vi "448benchmark1.vi"() -> ()   [LabVIEW 2017]
uses:
  user.lib/_NEVSTOP/Communicable State Machine(CSM)/_Support/Typedef/_CSM_GlobalLog_MSG.ctl
  user.lib/_NEVSTOP/Communicable State Machine(CSM)/_Support/Typedef/_CSM_Response Source Message.ctl
  user.lib/_NEVSTOP/Communicable State Machine(CSM)/_Support/Typedef/_CSM_GlobalLog_MSG_TYPE.ctl
  user.lib/_NEVSTOP/Communicable State Machine(CSM)/_Support/GlobalEvent/GEvt-Refs.ctl
  user.lib/_NEVSTOP/Communicable State Machine(CSM)/Communicable State Machine.lvlib
panel:
  out "inside 2":i32
  out "outside 2":i32
  out "inside":i32
  out "outside":i32
  out "unit (ms)":dbl[][](graph)
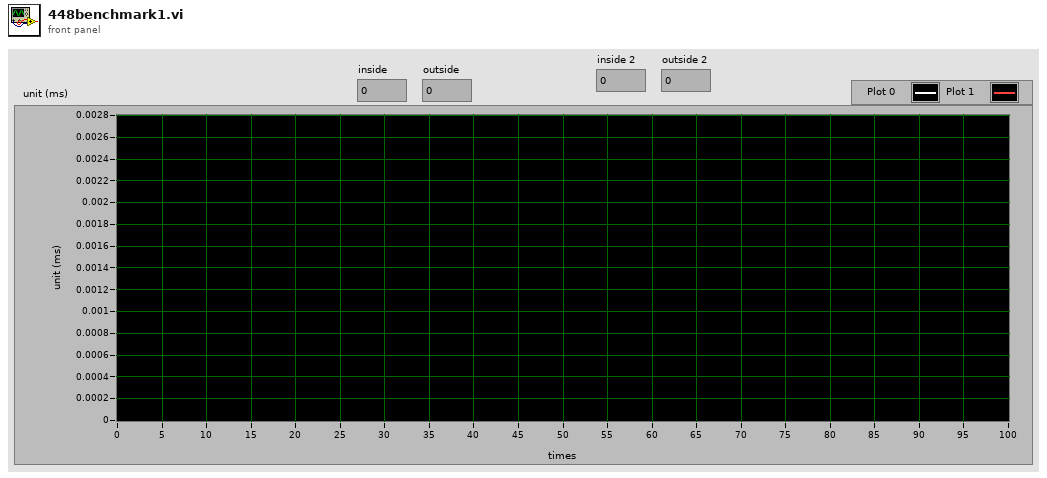
[diagram p1: front panel]
types:
  T1 = typedef "GEvt-Refs.ctl" = cluster{"Event":refnum<user-event>, "Queues":refnum<queue>[], "Valid":bool}
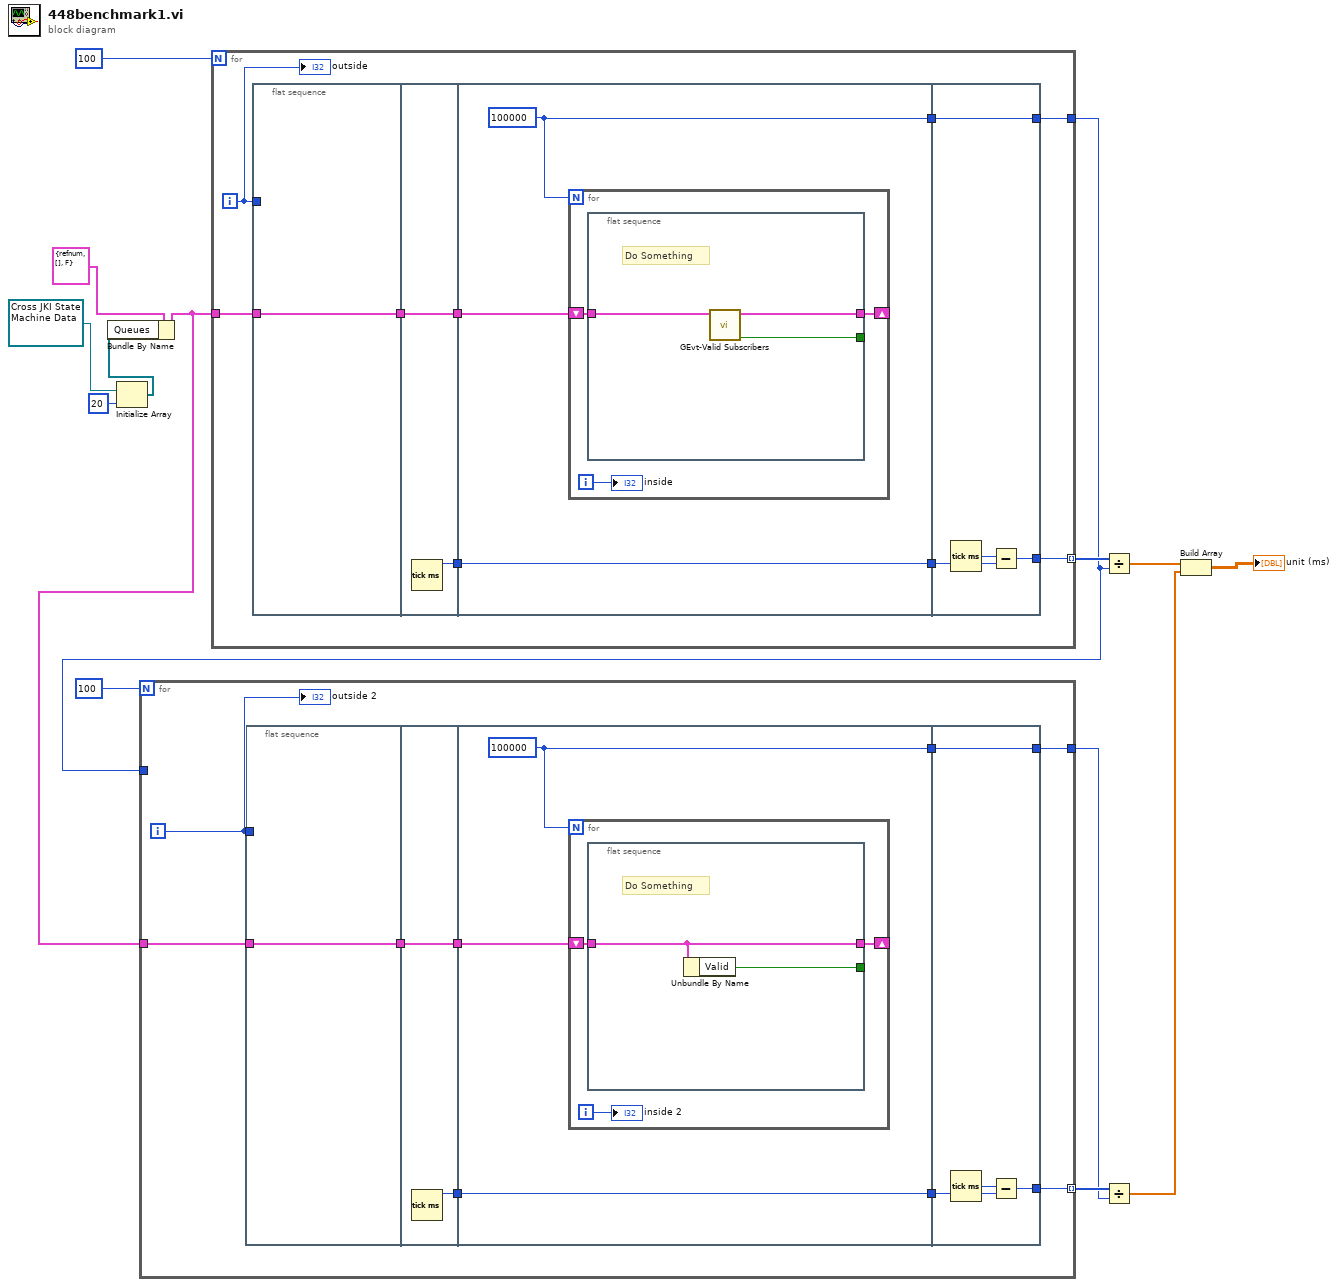
[diagram p0: block diagram]
diagram:
  n1 = Initialize Array(refnum<queue> refnum ("Queue"), 20 ("dimension size")) -> (w2:refnum<queue>[])
  n2 = Bundle By Name(cluster=T1 {"Event"=refnum, "Queues"=[], "Valid"=FALSE} ("CSM Global Log Event in"), "Queues"=w2) -> (w1:T1)
  n3 = for {
    N: 100 -> [_]
    tunnel: [w21] -> w14 mode=indexing
    tunnel: [w20] -> w6
    tunnel: w1 -> [w15]
    i -> [w18]
    n4 = flat-sequence {
      tunnel: w18 -> [_]
      tunnel: [w24] -> w16
      tunnel: w15 -> [w24]
      tunnel: [w26] -> w23
      tunnel: [w25] -> w17
      tunnel: w16 -> [w25]
      tunnel: w23 -> [w29]
      tunnel: [w29] -> w22
      tunnel: [w28] -> w19
      tunnel: w17 -> [w27]
      tunnel: w22 -> [w38]
      tunnel: [w37] -> w21
      tunnel: [w36] -> w20
      tunnel: w19 -> [w36]
      frame #0 {
      }
      frame #1 {
        n5 = Tick Count (ms)() -> (millisecond timer value=w26:u32)
      }
      frame #2 {
        w28 = 100000
        n6 = for {
          N: w28 -> [_]
          shift-right: [w30] -> _
          shift-left: w27 -> [w31]
          i -> [w32]
          n7 = flat-sequence {
            tunnel: w31 -> [w35]
            tunnel: [w34] -> _
            tunnel: [w33] -> w30
            frame #0 {
              # "Do Something"
              n8 = call "GEvt-Valid Subscribers.vi"("CSM Global Log Event in"=w35) -> ("Valid"=w34:bool, "CSM Global Log Event out"=w33:T1)  [unwired: 9 in]
            }
          }
          "inside" <- w32
        }
      }
      frame #3 {
        n9 = Tick Count (ms)() -> (millisecond timer value=w39:u32)
        n10 = Subtract(x=w39, y=w38) -> (x-y=w37:u32)
      }
    }
    "outside" <- w18
  }
  n11 = for {
    N: 100 -> [_]
    tunnel: [w46] -> w10 mode=indexing
    tunnel: [w45] -> w9
    tunnel: w6 -> [_]
    tunnel: w1 -> [w40]
    i -> [w43]
    n12 = flat-sequence {
      tunnel: w43 -> [_]
      tunnel: [w49] -> w41
      tunnel: w40 -> [w49]
      tunnel: [w51] -> w48
      tunnel: [w50] -> w42
      tunnel: w41 -> [w50]
      tunnel: w48 -> [w54]
      tunnel: [w54] -> w47
      tunnel: [w53] -> w44
      tunnel: w42 -> [w52]
      tunnel: w47 -> [w62]
      tunnel: [w61] -> w46
      tunnel: [w60] -> w45
      tunnel: w44 -> [w60]
      frame #0 {
      }
      frame #1 {
        n13 = Tick Count (ms)() -> (millisecond timer value=w51:u32)
      }
      frame #2 {
        w53 = 100000
        n14 = for {
          N: w53 -> [_]
          shift-right: [w55] -> _
          shift-left: w52 -> [w56]
          i -> [w57]
          n15 = flat-sequence {
            tunnel: w56 -> [w59]
            tunnel: [w58] -> _
            tunnel: [w59] -> w55
            frame #0 {
              # "Do Something"
              n16 = Unbundle By Name(w59) -> ("Valid"=w58:bool)
            }
          }
          "inside 2" <- w57
        }
      }
      frame #3 {
        n17 = Tick Count (ms)() -> (millisecond timer value=w63:u32)
        n18 = Subtract(x=w63, y=w62) -> (x-y=w61:u32)
      }
    }
    "outside 2" <- w43
  }
  n19 = Divide(x=w14, y=w6) -> (x/y=w13:dbl[])
  n20 = Divide(x=w10, y=w9) -> (x/y=w7:dbl[])
  n21 = Build Array(w13, w7) -> (→"unit (ms)":dbl[][])
